vi "Do.vi"(8 "error in (no error)":errorcluster, 10 "Actor in":refnum<class "Actor.lvclass">, 11 "StopTrigger Msg":refnum<class "StopTrigger Msg.lvclass">) -> (0 "error out":errorcluster, 2 "Actor out":refnum<class "Actor.lvclass">)   [LabVIEW 2019, in "PredictiveMaintenance.lvlib" / "StopTrigger Msg.lvclass"]
doc: "This VI delivers the message to the actor by calling the appropriate method(s) on the actor."
uses:
  StopTrigger Msg.lvclass
  PredictiveMaintenance/PredictiveMaintenance.lvclass
  C:/Program Files (x86)/National Instruments/LabVIEW 2019/vi.lib/ActorFramework/Actor/Actor.lvclass
  <vilib>/ActorFramework/Actor/Actor.lvclass
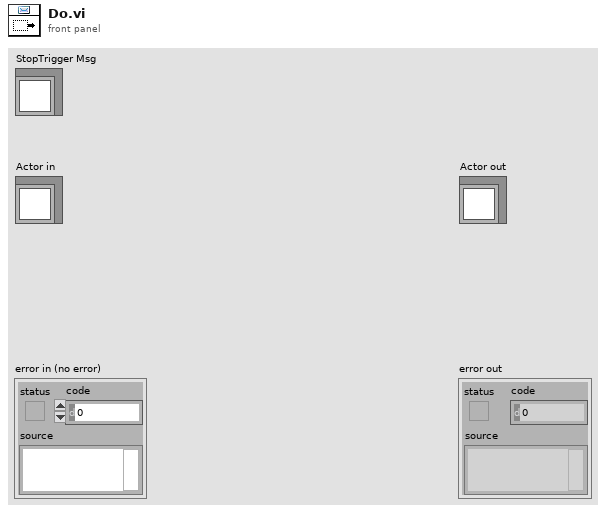
[diagram p1: front panel]
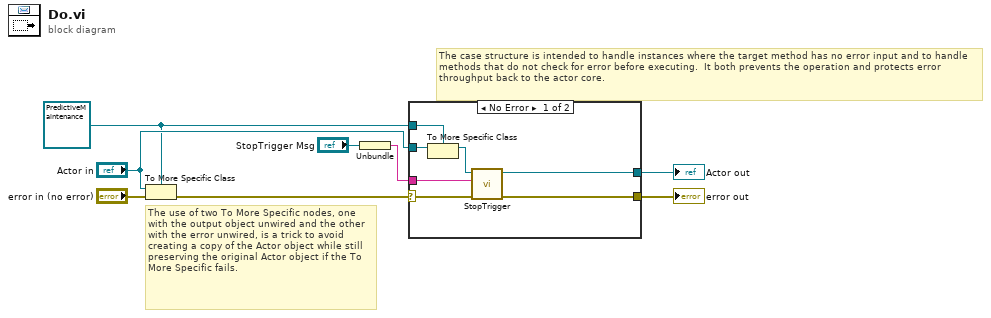
[diagram p0: block diagram]
diagram:
  w1 = refnum<class "PredictiveMaintenance.lvclass"> refnum ("PredictiveMaintenance.lvlib:PredictiveMaintenance.lvclass")
  # "The use of two To More Specific nodes, one with the output object unwired and the other with the error unwired, is a trick to avoid creating a copy of the Actor object while still preserving the original Actor object if the To More Specific fails."
  # "The case structure is intended to handle instances where the target method has no error input and to handle methods that do not check for error before executing.  It both prevents the operation and protects error throughput back to the actor core."
  n1 = To More Specific Class(target class=w1, reference="Actor in", error in="error in (no error)") -> (error out=w6:errorcluster)  [unwired: 1 out]
  n2 = Unbundle("StopTrigger Msg") -> (w2:string)
  n3 = case shown="No Error" w6 {
    selector: w6 -> [w11 w17]
    tunnel: [w10 w17] -> w5
    tunnel: [w9 w16] -> w4
    tunnel: "Actor in" -> [w15 w16]
    tunnel: w1 -> [w14 _]
    tunnel: w2 -> [w12 _]
    frame No Error {
      n4 = To More Specific Class(target class=w14, reference=w15) -> (specific class reference=w13:refnum<class "PredictiveMaintenance.lvclass">)  [unwired: 1 in, 1 out]
      n5 = call-dynamic "StopTrigger.vi"("error in (no error)"=w11, "trigger"=w12, "PredictiveMaintenance in"=w13) -> ("error out"=w10:errorcluster, "PredictiveMaintenance out"=w9:refnum<class "PredictiveMaintenance.lvclass">)  [unwired: 7 in]
    }
    frame Error {
      # "If type check fails, pass the original object out again."
    }
  }
  "error out" <- w5
  "Actor out" <- w4
